vi "PB-01 Write.vi"(0 "Device Inputs":dbl[](array[numeric]), 12 "PB-01 in":T1={"FIFO Indexes"={"Write"={"Clear Faults"=0, "ESTTL Setup"=[], "UEGO Control"={"UEGO1Enable"=-1, "UEGO2Enable"=-1, "UEGO1Range"=-1, "UEGO2Range"=-1, "FilterCutoff (Hz)"=-1}}, "Read"={"UEGO Sensor Results"={"UEGO1Lambda"=-1, "UEGO1Phi"=-1, "UEGO1AFRatio"=-1, "UEGO1Ip (mA)"=-1, "UEGO2Lambda"=-1, "UEGO2Phi"=-1, "UEGO2AFRatio"=-1, "UEGO2Ip (mA)"=-1}, "UEGO Temperature (C)"={"UEGO1Temp (C)"=-1, "UEGO2Temp (C)"=-1, "UEGO1Hot"=-1, "UEGO2Hot"=-1}, "UEGO Diagnostics"={"UEGO1SensorFault"=-1, "UEGO2SensorFault"=-1, "UEGO1HeaterFault"=-1, "UEGO2HeaterFault"=-1, "UEGOFuseStatus"=-1, "Battery (V)"=-1, "LSUType"=-1}}}, "Settings"={"VR-Hall Mode Select"=[enum."VR Adaptive Arm", enum."VR Adaptive Arm", enum."VR Adaptive Arm", enum."VR Adaptive Arm", enum."VR Adaptive Arm"], "VR-Hall Arming Threshold [V]"=[0.0, 0.0, 0.0, 0.0, 0.0], "ESTTL Command Enabled"=FALSE}} {"FIFO Indexes"."Read"."UEGO Diagnostics"."LSUType" format="%02.0f"; "FIFO Indexes"."Read"."UEGO Diagnostics"."UEGOFuseStatus" format="%02.0f"}) -> (4 "VR-Hall Mode Select":T3[](array[typedef])=[enum."VR Adaptive Arm", enum."VR Adaptive Arm", enum."VR Adaptive Arm", enum."VR Adaptive Arm", enum."VR Adaptive Arm"], 6 "VR-Hall Arming/Threshold [V]":dbl[](array[numeric]), 8 "SensorControl":T7={"UEGO1Enable"=FALSE, "UEGO2Enable"=FALSE, "UEGO1Range"=FALSE, "UEGO2Range"=FALSE, "FilterCutoff (Hz)"=10.0}, 10 "Clear Faults":bool, 15 "ESTTL Setup":T4[](array[typedef])=[{"Mode"=enum."Off", "Polarity"=FALSE, "Frequency [Hz]"=0.0, "Duty Cycle [%]"=0.0, "TDC Offset [CAD]"=0.0, "Window Start [DBTDC]"=0.0, "Window End [DBTDC]"=0.0, "Angles"=[{"Enable"=FALSE, "Location [DBTDC]"=0.0, "Duration [s]"=0.0}, {"Enable"=FALSE, "Location [DBTDC]"=0.0, "Duration [s]"=0.0}, {"Enable"=FALSE, "Location [DBTDC]"=0.0, "Duration [s]"=0.0}, {"Enable"=FALSE, "Location [DBTDC]"=0.0, "Duration [s]"=0.0}], "Skip Fire"=FALSE, "Skip Fire Index"=0}, {"Mode"=enum."Off", "Polarity"=FALSE, "Frequency [Hz]"=0.0, "Duty Cycle [%]"=0.0, "TDC Offset [CAD]"=0.0, "Window Start [DBTDC]"=0.0, "Window End [DBTDC]"=0.0, "Angles"=[{"Enable"=FALSE, "Location [DBTDC]"=0.0, "Duration [s]"=0.0}, {"Enable"=FALSE, "Location [DBTDC]"=0.0, "Duration [s]"=0.0}, {"Enable"=FALSE, "Location [DBTDC]"=0.0, "Duration [s]"=0.0}, {"Enable"=FALSE, "Location [DBTDC]"=0.0, "Duration [s]"=0.0}], "Skip Fire"=FALSE, "Skip Fire Index"=0}, {"Mode"=enum."Off", "Polarity"=FALSE, "Frequency [Hz]"=0.0, "Duty Cycle [%]"=0.0, "TDC Offset [CAD]"=0.0, "Window Start [DBTDC]"=0.0, "Window End [DBTDC]"=0.0, "Angles"=[{"Enable"=FALSE, "Location [DBTDC]"=0.0, "Duration [s]"=0.0}, {"Enable"=FALSE, "Location [DBTDC]"=0.0, "Duration [s]"=0.0}, {"Enable"=FALSE, "Location [DBTDC]"=0.0, "Duration [s]"=0.0}, {"Enable"=FALSE, "Location [DBTDC]"=0.0, "Duration [s]"=0.0}], "Skip Fire"=FALSE, "Skip Fire Index"=0}, {"Mode"=enum."Off", "Polarity"=FALSE, "Frequency [Hz]"=0.0, "Duty Cycle [%]"=0.0, "TDC Offset [CAD]"=0.0, "Window Start [DBTDC]"=0.0, "Window End [DBTDC]"=0.0, "Angles"=[{"Enable"=FALSE, "Location [DBTDC]"=0.0, "Duration [s]"=0.0}, {"Enable"=FALSE, "Location [DBTDC]"=0.0, "Duration [s]"=0.0}, {"Enable"=FALSE, "Location [DBTDC]"=0.0, "Duration [s]"=0.0}, {"Enable"=FALSE, "Location [DBTDC]"=0.0, "Duration [s]"=0.0}], "Skip Fire"=FALSE, "Skip Fire Index"=0}, {"Mode"=enum."Off", "Polarity"=FALSE, "Frequency [Hz]"=0.0, "Duty Cycle [%]"=0.0, "TDC Offset [CAD]"=0.0, "Window Start [DBTDC]"=0.0, "Window End [DBTDC]"=0.0, "Angles"=[{"Enable"=FALSE, "Location [DBTDC]"=0.0, "Duration [s]"=0.0}, {"Enable"=FALSE, "Location [DBTDC]"=0.0, "Duration [s]"=0.0}, {"Enable"=FALSE, "Location [DBTDC]"=0.0, "Duration [s]"=0.0}, {"Enable"=FALSE, "Location [DBTDC]"=0.0, "Duration [s]"=0.0}], "Skip Fire"=FALSE, "Skip Fire Index"=0}, {"Mode"=enum."Off", "Polarity"=FALSE, "Frequency [Hz]"=0.0, "Duty Cycle [%]"=0.0, "TDC Offset [CAD]"=0.0, "Window Start [DBTDC]"=0.0, "Window End [DBTDC]"=0.0, "Angles"=[{"Enable"=FALSE, "Location [DBTDC]"=0.0, "Duration [s]"=0.0}, {"Enable"=FALSE, "Location [DBTDC]"=0.0, "Duration [s]"=0.0}, {"Enable"=FALSE, "Location [DBTDC]"=0.0, "Duration [s]"=0.0}, {"Enable"=FALSE, "Location [DBTDC]"=0.0, "Duration [s]"=0.0}], "Skip Fire"=FALSE, "Skip Fire Index"=0}, {"Mode"=enum."Off", "Polarity"=FALSE, "Frequency [Hz]"=0.0, "Duty Cycle [%]"=0.0, "TDC Offset [CAD]"=0.0, "Window Start [DBTDC]"=0.0, "Window End [DBTDC]"=0.0, "Angles"=[{"Enable"=FALSE, "Location [DBTDC]"=0.0, "Duration [s]"=0.0}, {"Enable"=FALSE, "Location [DBTDC]"=0.0, "Duration [s]"=0.0}, {"Enable"=FALSE, "Location [DBTDC]"=0.0, "Duration [s]"=0.0}, {"Enable"=FALSE, "Location [DBTDC]"=0.0, "Duration [s]"=0.0}], "Skip Fire"=FALSE, "Skip Fire Index"=0}, {"Mode"=enum."Off", "Polarity"=FALSE, "Frequency [Hz]"=0.0, "Duty Cycle [%]"=0.0, "TDC Offset [CAD]"=0.0, "Window Start [DBTDC]"=0.0, "Window End [DBTDC]"=0.0, "Angles"=[{"Enable"=FALSE, "Location [DBTDC]"=0.0, "Duration [s]"=0.0}, {"Enable"=FALSE, "Location [DBTDC]"=0.0, "Duration [s]"=0.0}, {"Enable"=FALSE, "Location [DBTDC]"=0.0, "Duration [s]"=0.0}, {"Enable"=FALSE, "Location [DBTDC]"=0.0, "Duration [s]"=0.0}], "Skip Fire"=FALSE, "Skip Fire Index"=0}, {"Mode"=enum."Off", "Polarity"=FALSE, "Frequency [Hz]"=0.0, "Duty Cycle [%]"=0.0, "TDC Offset [CAD]"=0.0, "Window Start [DBTDC]"=0.0, "Window End [DBTDC]"=0.0, "Angles"=[{"Enable"=FALSE, "Location [DBTDC]"=0.0, "Duration [s]"=0.0}, {"Enable"=FALSE, "Location [DBTDC]"=0.0, "Duration [s]"=0.0}, {"Enable"=FALSE, "Location [DBTDC]"=0.0, "Duration [s]"=0.0}, {"Enable"=FALSE, "Location [DBTDC]"=0.0, "Duration [s]"=0.0}], "Skip Fire"=FALSE, "Skip Fire Index"=0}, {"Mode"=enum."Off", "Polarity"=FALSE, "Frequency [Hz]"=0.0, "Duty Cycle [%]"=0.0, "TDC Offset [CAD]"=0.0, "Window Start [DBTDC]"=0.0, "Window End [DBTDC]"=0.0, "Angles"=[{"Enable"=FALSE, "Location [DBTDC]"=0.0, "Duration [s]"=0.0}, {"Enable"=FALSE, "Location [DBTDC]"=0.0, "Duration [s]"=0.0}, {"Enable"=FALSE, "Location [DBTDC]"=0.0, "Duration [s]"=0.0}, {"Enable"=FALSE, "Location [DBTDC]"=0.0, "Duration [s]"=0.0}], "Skip Fire"=FALSE, "Skip Fire Index"=0}, {"Mode"=enum."Off", "Polarity"=FALSE, "Frequency [Hz]"=0.0, "Duty Cycle [%]"=0.0, "TDC Offset [CAD]"=0.0, "Window Start [DBTDC]"=0.0, "Window End [DBTDC]"=0.0, "Angles"=[{"Enable"=FALSE, "Location [DBTDC]"=0.0, "Duration [s]"=0.0}, {"Enable"=FALSE, "Location [DBTDC]"=0.0, "Duration [s]"=0.0}, {"Enable"=FALSE, "Location [DBTDC]"=0.0, "Duration [s]"=0.0}, {"Enable"=FALSE, "Location [DBTDC]"=0.0, "Duration [s]"=0.0}], "Skip Fire"=FALSE, "Skip Fire Index"=0}, {"Mode"=enum."Off", "Polarity"=FALSE, "Frequency [Hz]"=0.0, "Duty Cycle [%]"=0.0, "TDC Offset [CAD]"=0.0, "Window Start [DBTDC]"=0.0, "Window End [DBTDC]"=0.0, "Angles"=[{"Enable"=FALSE, "Location [DBTDC]"=0.0, "Duration [s]"=0.0}, {"Enable"=FALSE, "Location [DBTDC]"=0.0, "Duration [s]"=0.0}, {"Enable"=FALSE, "Location [DBTDC]"=0.0, "Duration [s]"=0.0}, {"Enable"=FALSE, "Location [DBTDC]"=0.0, "Duration [s]"=0.0}], "Skip Fire"=FALSE, "Skip Fire Index"=0}, {"Mode"=enum."Off", "Polarity"=FALSE, "Frequency [Hz]"=0.0, "Duty Cycle [%]"=0.0, "TDC Offset [CAD]"=0.0, "Window Start [DBTDC]"=0.0, "Window End [DBTDC]"=0.0, "Angles"=[{"Enable"=FALSE, "Location [DBTDC]"=0.0, "Duration [s]"=0.0}, {"Enable"=FALSE, "Location [DBTDC]"=0.0, "Duration [s]"=0.0}, {"Enable"=FALSE, "Location [DBTDC]"=0.0, "Duration [s]"=0.0}, {"Enable"=FALSE, "Location [DBTDC]"=0.0, "Duration [s]"=0.0}], "Skip Fire"=FALSE, "Skip Fire Index"=0}, {"Mode"=enum."Off", "Polarity"=FALSE, "Frequency [Hz]"=0.0, "Duty Cycle [%]"=0.0, "TDC Offset [CAD]"=0.0, "Window Start [DBTDC]"=0.0, "Window End [DBTDC]"=0.0, "Angles"=[{"Enable"=FALSE, "Location [DBTDC]"=0.0, "Duration [s]"=0.0}, {"Enable"=FALSE, "Location [DBTDC]"=0.0, "Duration [s]"=0.0}, {"Enable"=FALSE, "Location [DBTDC]"=0.0, "Duration [s]"=0.0}, {"Enable"=FALSE, "Location [DBTDC]"=0.0, "Duration [s]"=0.0}], "Skip Fire"=FALSE, "Skip Fire Index"=0}, {"Mode"=enum."Off", "Polarity"=FALSE, "Frequency [Hz]"=0.0, "Duty Cycle [%]"=0.0, "TDC Offset [CAD]"=0.0, "Window Start [DBTDC]"=0.0, "Window End [DBTDC]"=0.0, "Angles"=[{"Enable"=FALSE, "Location [DBTDC]"=0.0, "Duration [s]"=0.0}, {"Enable"=FALSE, "Location [DBTDC]"=0.0, "Duration [s]"=0.0}, {"Enable"=FALSE, "Location [DBTDC]"=0.0, "Duration [s]"=0.0}, {"Enable"=FALSE, "Location [DBTDC]"=0.0, "Duration [s]"=0.0}], "Skip Fire"=FALSE, "Skip Fire Index"=0}, {"Mode"=enum."Off", "Polarity"=FALSE, "Frequency [Hz]"=0.0, "Duty Cycle [%]"=0.0, "TDC Offset [CAD]"=0.0, "Window Start [DBTDC]"=0.0, "Window End [DBTDC]"=0.0, "Angles"=[{"Enable"=FALSE, "Location [DBTDC]"=0.0, "Duration [s]"=0.0}, {"Enable"=FALSE, "Location [DBTDC]"=0.0, "Duration [s]"=0.0}, {"Enable"=FALSE, "Location [DBTDC]"=0.0, "Duration [s]"=0.0}, {"Enable"=FALSE, "Location [DBTDC]"=0.0, "Duration [s]"=0.0}], "Skip Fire"=FALSE, "Skip Fire Index"=0}] {"Skip Fire Index" max=7; "Angles"."Duration [s]" format="%#_3p"; "Frequency [Hz]" format="%#_3p"})   [LabVIEW 2015]
uses:
  <vilib>/Powertrain Controls/Device Drivers/VR-Hall/RevC/Real-Time/Support/Vr_Hall_mode_control_revc.ctl
  <vilib>/Powertrain Controls/Device Drivers/DCM/ESTTL/RT/Setup.ctl
  <vilib>/Powertrain Controls/Device Drivers/DCM/ESTTL/FPGA/Mode.ctl
  <vilib>/Powertrain Controls/Device Drivers/DCM/ESTTL/RT/Angle Control.ctl
  DCM-NIVS-RT/PB-01.ctl
  DCM-NIVS-RT/ESTTL Setup Indexes.ctl
  <vilib>/Powertrain Controls/Device Drivers/DCM/ESTTL/RT/DCM - RT - ESTTL.lvlib
  <vilib>/Powertrain Controls/Device Drivers/DCM/ESTTL/FPGA/DCM - FPGA - ESTTL.lvlib
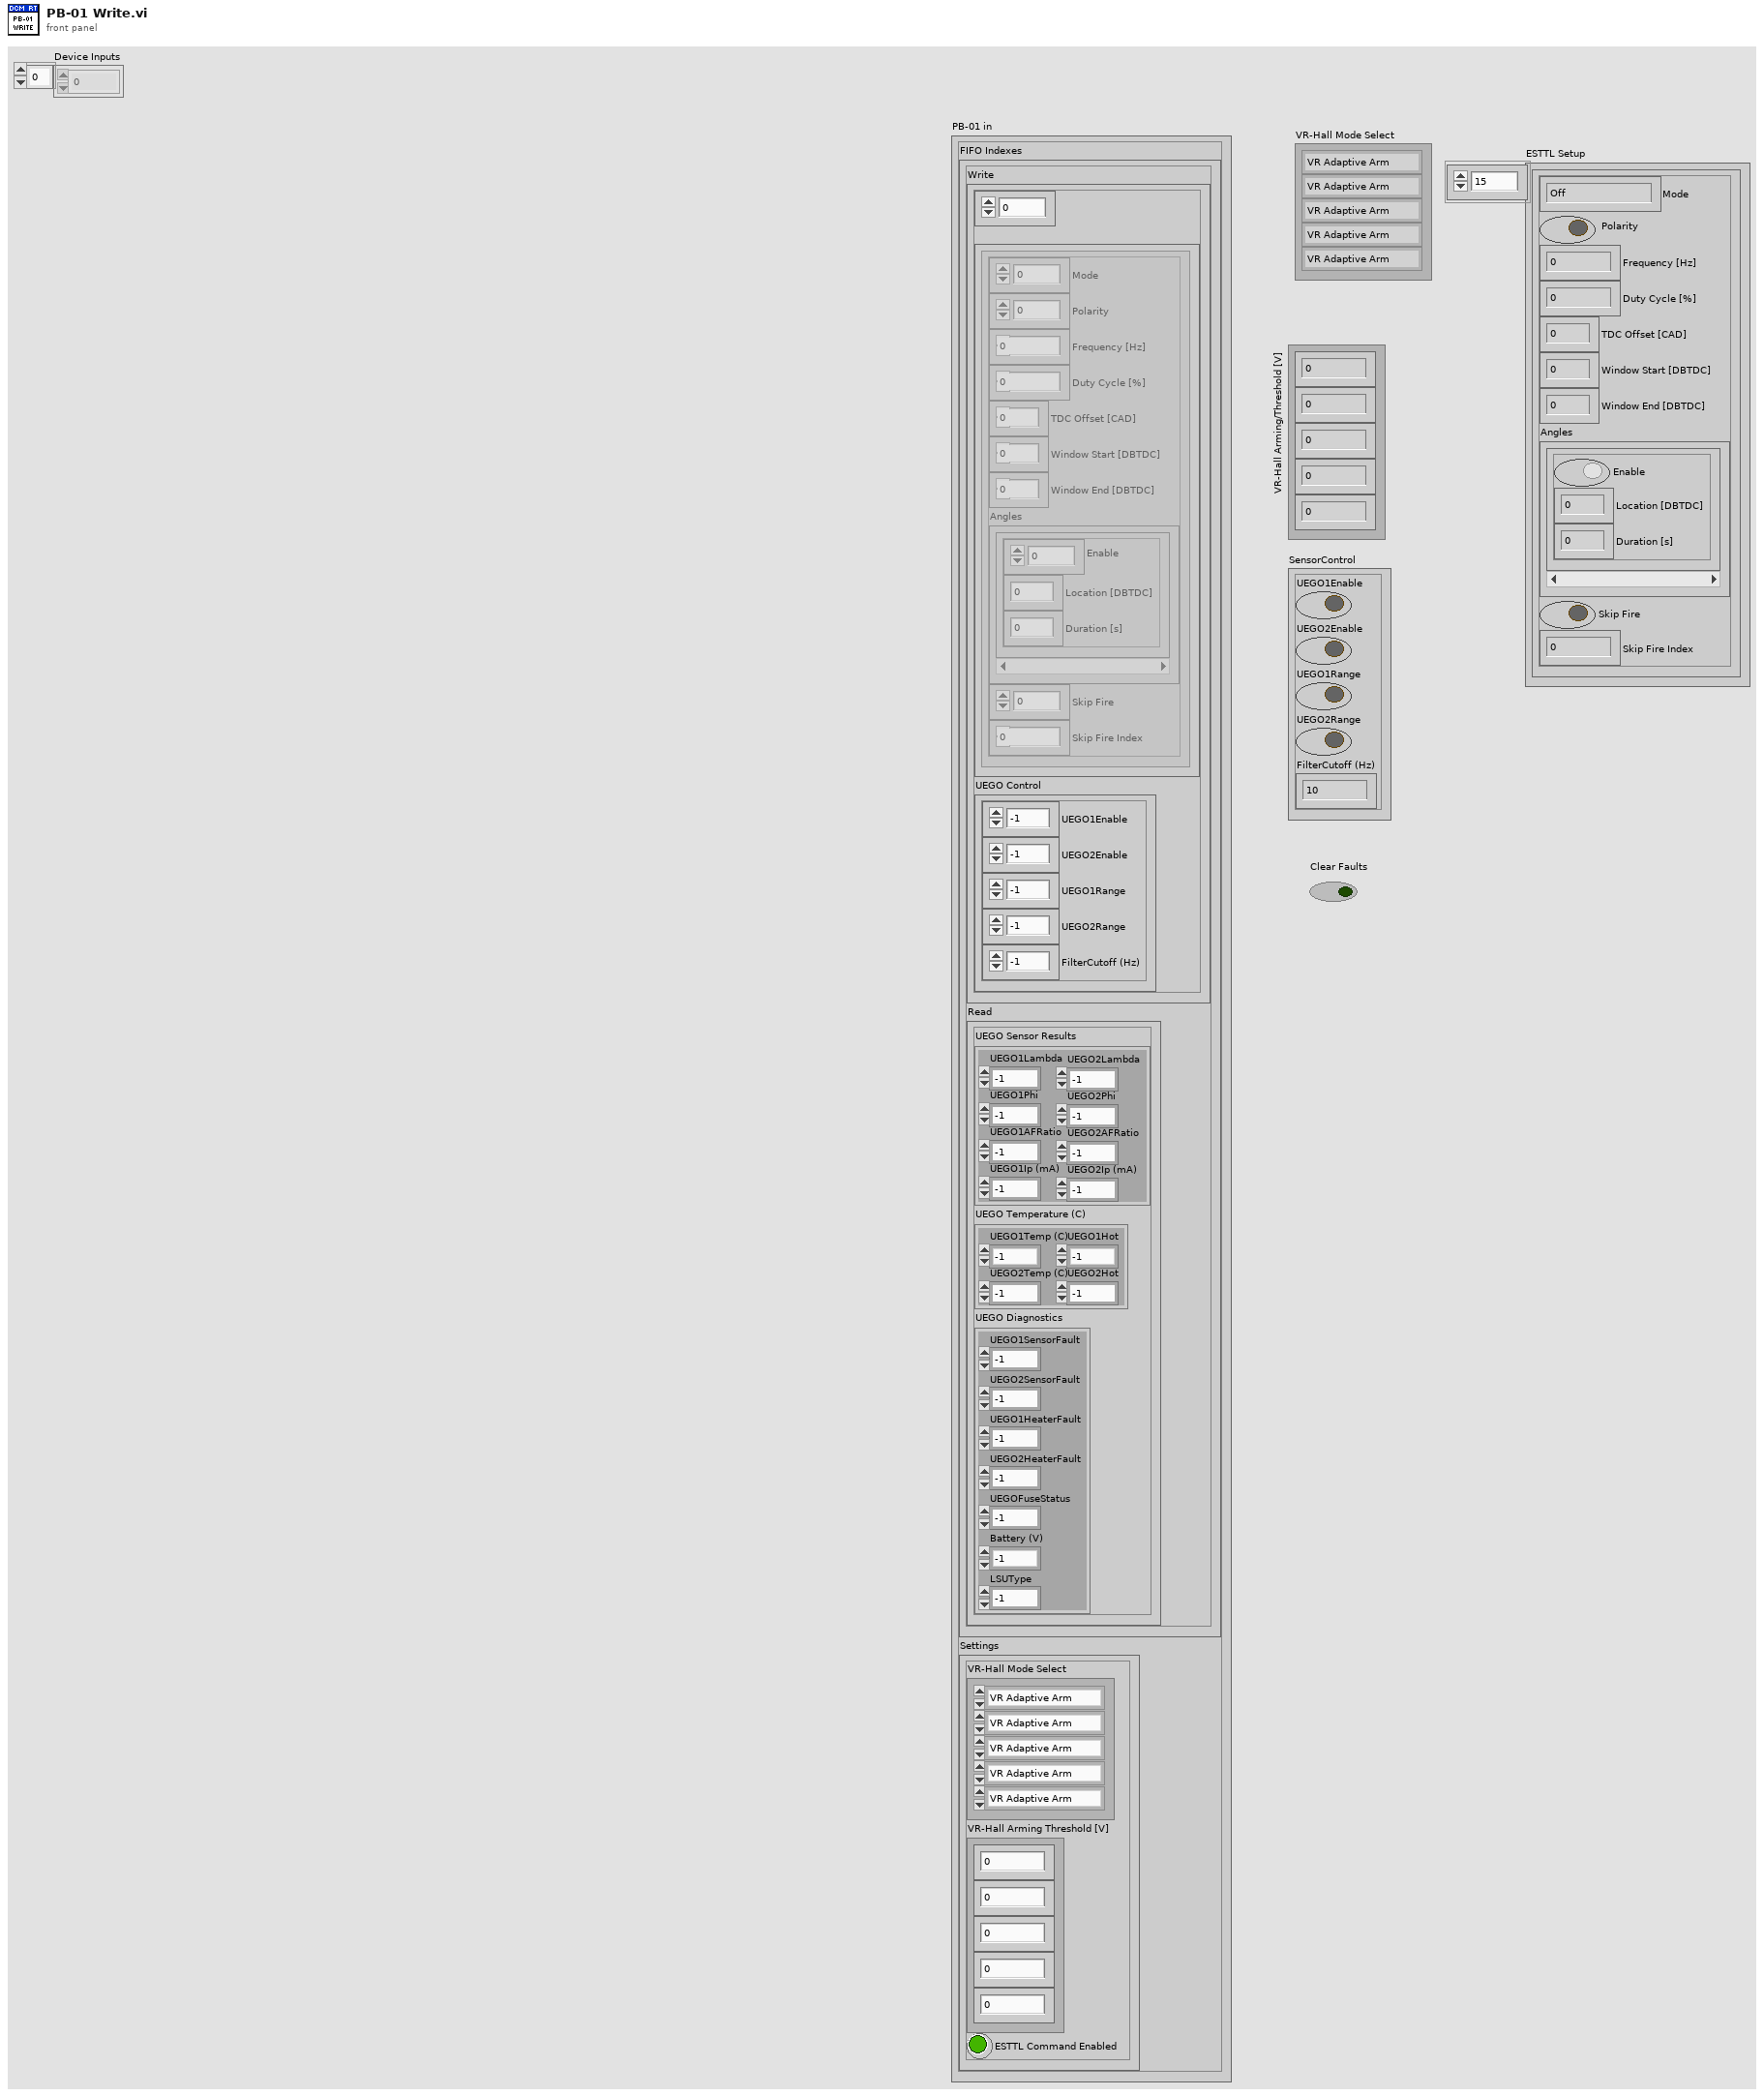
[diagram p1: front panel]
types:
  T1 = typedef "PB-01.ctl" = cluster{"FIFO Indexes":cluster{"Write":cluster{"Clear Faults":i32, "ESTTL Setup":T2[], "UEGO Control":cluster{"UEGO1Enable":i32, "UEGO2Enable":i32, "UEGO1Range":i32, "UEGO2Range":i32, "FilterCutoff (Hz)":i32}}, "Read":cluster{"UEGO Sensor Results":cluster{"UEGO1Lambda":i32, "UEGO1Phi":i32, "UEGO1AFRatio":i32, "UEGO1Ip (mA)":i32, "UEGO2Lambda":i32, "UEGO2Phi":i32, "UEGO2AFRatio":i32, "UEGO2Ip (mA)":i32}, "UEGO Temperature (C)":cluster{"UEGO1Temp (C)":i32, "UEGO2Temp (C)":i32, "UEGO1Hot":i32, "UEGO2Hot":i32}, "UEGO Diagnostics":cluster{"UEGO1SensorFault":i32, "UEGO2SensorFault":i32, "UEGO1HeaterFault":i32, "UEGO2HeaterFault":i32, "UEGOFuseStatus":i32, "Battery (V)":i32, "LSUType":i32}}}, "Settings":cluster{"VR-Hall Mode Select":T3[], "VR-Hall Arming Threshold [V]":dbl[], "ESTTL Command Enabled":bool}}
  T2 = typedef "ESTTL Setup Indexes.ctl" = cluster{"Mode":i32, "Polarity":i32, "Frequency [Hz]":i32, "Duty Cycle [%]":i32, "TDC Offset [CAD]":i32, "Window Start [DBTDC]":i32, "Window End [DBTDC]":i32, "Angles":cluster{"Enable":i32, "Location [DBTDC]":i32, "Duration [s]":i32}[], "Skip Fire":i32, "Skip Fire Index":i32}
  T3 = typedef "Vr_Hall_mode_control_revc.ctl" = enum32{"VR Adaptive Arm", "VR Manual Arm", "Hall", "Hall w/ Pull-up"}
  T4 = typedef "DCM - RT - ESTTL.lvlib/Setup.ctl" = cluster{"Mode":T5, "Polarity":bool, "Frequency [Hz]":sgl, "Duty Cycle [%]":sgl, "TDC Offset [CAD]":sgl, "Window Start [DBTDC]":sgl, "Window End [DBTDC]":sgl, "Angles":T6[], "Skip Fire":bool, "Skip Fire Index":u8}
  T5 = typedef "DCM - FPGA - ESTTL.lvlib/Mode.ctl" = enum8{"Off", "Pulse Width Modulation", "Engine Position Tracking"}
  T6 = typedef "DCM - RT - ESTTL.lvlib/Angle Control.ctl" = cluster{"Enable":bool, "Location [DBTDC]":sgl, "Duration [s]":sgl}
  T7 = cluster{"UEGO1Enable":bool, "UEGO2Enable":bool, "UEGO1Range":bool, "UEGO2Range":bool, "FilterCutoff (Hz)":dbl}
  T8 = cluster{"UEGO1Enable":i32, "UEGO2Enable":i32, "UEGO1Range":i32, "UEGO2Range":i32, "FilterCutoff (Hz)":i32}
  T9 = cluster{"Enable":i32, "Location [DBTDC]":i32, "Duration [s]":i32}[]
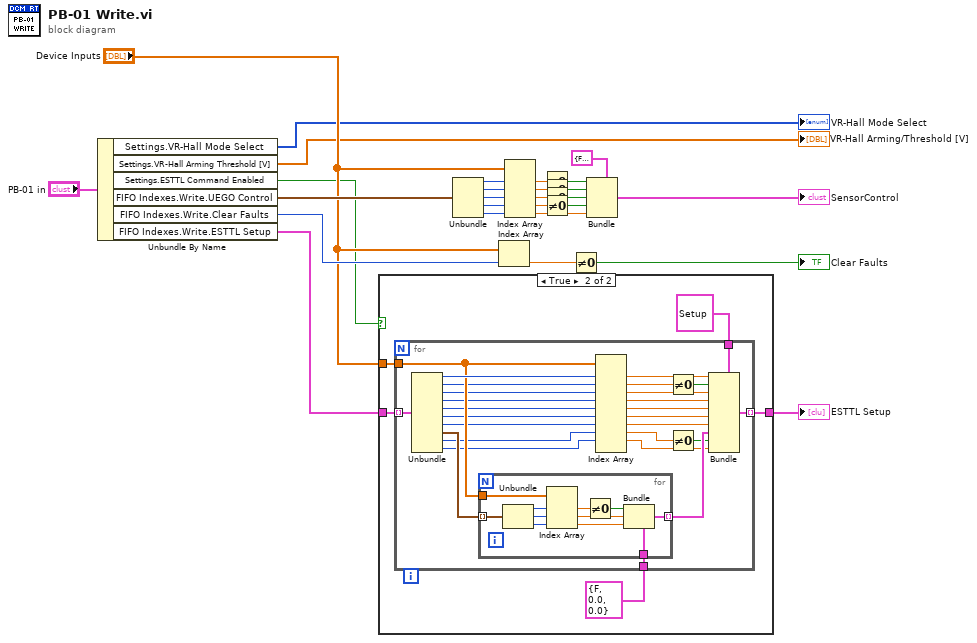
[diagram p0: block diagram]
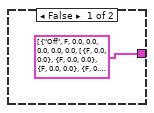
[diagram p2: hidden frame]
diagram:
  n1 = Unbundle By Name("PB-01 in") -> ("Settings.VR-Hall Mode Select"=→"VR-Hall Mode Select":T3[], "Settings.VR-Hall Arming Threshold [V]"=→"VR-Hall Arming/Threshold [V]":dbl[], "Settings.ESTTL Command Enabled"=w1:bool, "FIFO Indexes.Write.UEGO Control"=w23:T8, "FIFO Indexes.Write.Clear Faults"=w26:i32, "FIFO Indexes.Write.ESTTL Setup"=w27:T2[])
  n2 = case shown="True" w1 {
    tunnel: w27 -> [_ w33]
    tunnel: [T4[] [{"Mode"=enum."Off", "Polarity"=FALSE, "Frequency [Hz]"=0.0, "Duty Cycle [%]"=0.0, "TDC Offset [CAD]"=0.0, "Window Start [DBTDC]"=0.0, "Window End [DBTDC]"=0.0, "Angles"=[{"Enable"=FALSE, "Location [DBTDC]"=0.0, "Duration [s]"=0.0}, {"Enable"=FALSE, "Location [DBTDC]"=0.0, "Duration [s]"=0.0}, {"Enable"=FALSE, "Location [DBTDC]"=0.0, "Duration [s]"=0.0}, {"Enable"=FALSE, "Location [DBTDC]"=0.0, "Duration [s]"=0.0}], "Skip Fire"=FALSE, "Skip Fire Index"=0}, {"Mode"=enum."Off", "Polarity"=FALSE, "Frequency [Hz]"=0.0, "Duty Cycle [%]"=0.0, "TDC Offset [CAD]"=0.0, "Window Start [DBTDC]"=0.0, "Window End [DBTDC]"=0.0, "Angles"=[{"Enable"=FALSE, "Location [DBTDC]"=0.0, "Duration [s]"=0.0}, {"Enable"=FALSE, "Location [DBTDC]"=0.0, "Duration [s]"=0.0}, {"Enable"=FALSE, "Location [DBTDC]"=0.0, "Duration [s]"=0.0}, {"Enable"=FALSE, "Location [DBTDC]"=0.0, "Duration [s]"=0.0}], "Skip Fire"=FALSE, "Skip Fire Index"=0}, {"Mode"=enum."Off", "Polarity"=FALSE, "Frequency [Hz]"=0.0, "Duty Cycle [%]"=0.0, "TDC Offset [CAD]"=0.0, "Window Start [DBTDC]"=0.0, "Window End [DBTDC]"=0.0, "Angles"=[{"Enable"=FALSE, "Location [DBTDC]"=0.0, "Duration [s]"=0.0}, {"Enable"=FALSE, "Location [DBTDC]"=0.0, "Duration [s]"=0.0}, {"Enable"=FALSE, "Location [DBTDC]"=0.0, "Duration [s]"=0.0}, {"Enable"=FALSE, "Location [DBTDC]"=0.0, "Duration [s]"=0.0}], "Skip Fire"=FALSE, "Skip Fire Index"=0}, {"Mode"=enum."Off", "Polarity"=FALSE, "Frequency [Hz]"=0.0, "Duty Cycle [%]"=0.0, "TDC Offset [CAD]"=0.0, "Window Start [DBTDC]"=0.0, "Window End [DBTDC]"=0.0, "Angles"=[{"Enable"=FALSE, "Location [DBTDC]"=0.0, "Duration [s]"=0.0}, {"Enable"=FALSE, "Location [DBTDC]"=0.0, "Duration [s]"=0.0}, {"Enable"=FALSE, "Location [DBTDC]"=0.0, "Duration [s]"=0.0}, {"Enable"=FALSE, "Location [DBTDC]"=0.0, "Duration [s]"=0.0}], "Skip Fire"=FALSE, "Skip Fire Index"=0}, {"Mode"=enum."Off", "Polarity"=FALSE, "Frequency [Hz]"=0.0, "Duty Cycle [%]"=0.0, "TDC Offset [CAD]"=0.0, "Window Start [DBTDC]"=0.0, "Window End [DBTDC]"=0.0, "Angles"=[{"Enable"=FALSE, "Location [DBTDC]"=0.0, "Duration [s]"=0.0}, {"Enable"=FALSE, "Location [DBTDC]"=0.0, "Duration [s]"=0.0}, {"Enable"=FALSE, "Location [DBTDC]"=0.0, "Duration [s]"=0.0}, {"Enable"=FALSE, "Location [DBTDC]"=0.0, "Duration [s]"=0.0}], "Skip Fire"=FALSE, "Skip Fire Index"=0}, {"Mode"=enum."Off", "Polarity"=FALSE, "Frequency [Hz]"=0.0, "Duty Cycle [%]"=0.0, "TDC Offset [CAD]"=0.0, "Window Start [DBTDC]"=0.0, "Window End [DBTDC]"=0.0, "Angles"=[{"Enable"=FALSE, "Location [DBTDC]"=0.0, "Duration [s]"=0.0}, {"Enable"=FALSE, "Location [DBTDC]"=0.0, "Duration [s]"=0.0}, {"Enable"=FALSE, "Location [DBTDC]"=0.0, "Duration [s]"=0.0}, {"Enable"=FALSE, "Location [DBTDC]"=0.0, "Duration [s]"=0.0}], "Skip Fire"=FALSE, "Skip Fire Index"=0}, {"Mode"=enum."Off", "Polarity"=FALSE, "Frequency [Hz]"=0.0, "Duty Cycle [%]"=0.0, "TDC Offset [CAD]"=0.0, "Window Start [DBTDC]"=0.0, "Window End [DBTDC]"=0.0, "Angles"=[{"Enable"=FALSE, "Location [DBTDC]"=0.0, "Duration [s]"=0.0}, {"Enable"=FALSE, "Location [DBTDC]"=0.0, "Duration [s]"=0.0}, {"Enable"=FALSE, "Location [DBTDC]"=0.0, "Duration [s]"=0.0}, {"Enable"=FALSE, "Location [DBTDC]"=0.0, "Duration [s]"=0.0}], "Skip Fire"=FALSE, "Skip Fire Index"=0}, {"Mode"=enum."Off", "Polarity"=FALSE, "Frequency [Hz]"=0.0, "Duty Cycle [%]"=0.0, "TDC Offset [CAD]"=0.0, "Window Start [DBTDC]"=0.0, "Window End [DBTDC]"=0.0, "Angles"=[{"Enable"=FALSE, "Location [DBTDC]"=0.0, "Duration [s]"=0.0}, {"Enable"=FALSE, "Location [DBTDC]"=0.0, "Duration [s]"=0.0}, {"Enable"=FALSE, "Location [DBTDC]"=0.0, "Duration [s]"=0.0}, {"Enable"=FALSE, "Location [DBTDC]"=0.0, "Duration [s]"=0.0}], "Skip Fire"=FALSE, "Skip Fire Index"=0}, {"Mode"=enum."Off", "Polarity"=FALSE, "Frequency [Hz]"=0.0, "Duty Cycle [%]"=0.0, "TDC Offset [CAD]"=0.0, "Window Start [DBTDC]"=0.0, "Window End [DBTDC]"=0.0, "Angles"=[{"Enable"=FALSE, "Location [DBTDC]"=0.0, "Duration [s]"=0.0}, {"Enable"=FALSE, "Location [DBTDC]"=0.0, "Duration [s]"=0.0}, {"Enable"=FALSE, "Location [DBTDC]"=0.0, "Duration [s]"=0.0}, {"Enable"=FALSE, "Location [DBTDC]"=0.0, "Duration [s]"=0.0}], "Skip Fire"=FALSE, "Skip Fire Index"=0}, {"Mode"=enum."Off", "Polarity"=FALSE, "Frequency [Hz]"=0.0, "Duty Cycle [%]"=0.0, "TDC Offset [CAD]"=0.0, "Window Start [DBTDC]"=0.0, "Window End [DBTDC]"=0.0, "Angles"=[{"Enable"=FALSE, "Location [DBTDC]"=0.0, "Duration [s]"=0.0}, {"Enable"=FALSE, "Location [DBTDC]"=0.0, "Duration [s]"=0.0}, {"Enable"=FALSE, "Location [DBTDC]"=0.0, "Duration [s]"=0.0}, {"Enable"=FALSE, "Location [DBTDC]"=0.0, "Duration [s]"=0.0}], "Skip Fire"=FALSE, "Skip Fire Index"=0}, {"Mode"=enum."Off", "Polarity"=FALSE, "Frequency [Hz]"=0.0, "Duty Cycle [%]"=0.0, "TDC Offset [CAD]"=0.0, "Window Start [DBTDC]"=0.0, "Window End [DBTDC]"=0.0, "Angles"=[{"Enable"=FALSE, "Location [DBTDC]"=0.0, "Duration [s]"=0.0}, {"Enable"=FALSE, "Location [DBTDC]"=0.0, "Duration [s]"=0.0}, {"Enable"=FALSE, "Location [DBTDC]"=0.0, "Duration [s]"=0.0}, {"Enable"=FALSE, "Location [DBTDC]"=0.0, "Duration [s]"=0.0}], "Skip Fire"=FALSE, "Skip Fire Index"=0}, {"Mode"=enum."Off", "Polarity"=FALSE, "Frequency [Hz]"=0.0, "Duty Cycle [%]"=0.0, "TDC Offset [CAD]"=0.0, "Window Start [DBTDC]"=0.0, "Window End [DBTDC]"=0.0, "Angles"=[{"Enable"=FALSE, "Location [DBTDC]"=0.0, "Duration [s]"=0.0}, {"Enable"=FALSE, "Location [DBTDC]"=0.0, "Duration [s]"=0.0}, {"Enable"=FALSE, "Location [DBTDC]"=0.0, "Duration [s]"=0.0}, {"Enable"=FALSE, "Location [DBTDC]"=0.0, "Duration [s]"=0.0}], "Skip Fire"=FALSE, "Skip Fire Index"=0}, {"Mode"=enum."Off", "Polarity"=FALSE, "Frequency [Hz]"=0.0, "Duty Cycle [%]"=0.0, "TDC Offset [CAD]"=0.0, "Window Start [DBTDC]"=0.0, "Window End [DBTDC]"=0.0, "Angles"=[{"Enable"=FALSE, "Location [DBTDC]"=0.0, "Duration [s]"=0.0}, {"Enable"=FALSE, "Location [DBTDC]"=0.0, "Duration [s]"=0.0}, {"Enable"=FALSE, "Location [DBTDC]"=0.0, "Duration [s]"=0.0}, {"Enable"=FALSE, "Location [DBTDC]"=0.0, "Duration [s]"=0.0}], "Skip Fire"=FALSE, "Skip Fire Index"=0}, {"Mode"=enum."Off", "Polarity"=FALSE, "Frequency [Hz]"=0.0, "Duty Cycle [%]"=0.0, "TDC Offset [CAD]"=0.0, "Window Start [DBTDC]"=0.0, "Window End [DBTDC]"=0.0, "Angles"=[{"Enable"=FALSE, "Location [DBTDC]"=0.0, "Duration [s]"=0.0}, {"Enable"=FALSE, "Location [DBTDC]"=0.0, "Duration [s]"=0.0}, {"Enable"=FALSE, "Location [DBTDC]"=0.0, "Duration [s]"=0.0}, {"Enable"=FALSE, "Location [DBTDC]"=0.0, "Duration [s]"=0.0}], "Skip Fire"=FALSE, "Skip Fire Index"=0}, {"Mode"=enum."Off", "Polarity"=FALSE, "Frequency [Hz]"=0.0, "Duty Cycle [%]"=0.0, "TDC Offset [CAD]"=0.0, "Window Start [DBTDC]"=0.0, "Window End [DBTDC]"=0.0, "Angles"=[{"Enable"=FALSE, "Location [DBTDC]"=0.0, "Duration [s]"=0.0}, {"Enable"=FALSE, "Location [DBTDC]"=0.0, "Duration [s]"=0.0}, {"Enable"=FALSE, "Location [DBTDC]"=0.0, "Duration [s]"=0.0}, {"Enable"=FALSE, "Location [DBTDC]"=0.0, "Duration [s]"=0.0}], "Skip Fire"=FALSE, "Skip Fire Index"=0}, {"Mode"=enum."Off", "Polarity"=FALSE, "Frequency [Hz]"=0.0, "Duty Cycle [%]"=0.0, "TDC Offset [CAD]"=0.0, "Window Start [DBTDC]"=0.0, "Window End [DBTDC]"=0.0, "Angles"=[{"Enable"=FALSE, "Location [DBTDC]"=0.0, "Duration [s]"=0.0}, {"Enable"=FALSE, "Location [DBTDC]"=0.0, "Duration [s]"=0.0}, {"Enable"=FALSE, "Location [DBTDC]"=0.0, "Duration [s]"=0.0}, {"Enable"=FALSE, "Location [DBTDC]"=0.0, "Duration [s]"=0.0}], "Skip Fire"=FALSE, "Skip Fire Index"=0}] ("ESTTL Setup") w30] -> w5
    tunnel: "Device Inputs" -> [_ w29]
    frame False {
    }
    frame True {
      n3 = for {
        tunnel: w33 -> [w60] mode=indexing
        tunnel: w29 -> [w57]
        tunnel: T6 {"Enable"=FALSE, "Location [DBTDC]"=0.0, "Duration [s]"=0.0} ("Injection Control") -> [w48]
        tunnel: T4 {"Mode"=enum."Off", "Polarity"=FALSE, "Frequency [Hz]"=0.0, "Duty Cycle [%]"=0.0, "TDC Offset [CAD]"=0.0, "Window Start [DBTDC]"=0.0, "Window End [DBTDC]"=0.0, "Angles"=[{"Enable"=FALSE, "Location [DBTDC]"=0.0, "Duration [s]"=0.0}, {"Enable"=FALSE, "Location [DBTDC]"=0.0, "Duration [s]"=0.0}, {"Enable"=FALSE, "Location [DBTDC]"=0.0, "Duration [s]"=0.0}, {"Enable"=FALSE, "Location [DBTDC]"=0.0, "Duration [s]"=0.0}], "Skip Fire"=FALSE, "Skip Fire Index"=0} ("DCM - RevB - RT - ESTTL.lvlib:Setup") -> [w35]
        tunnel: [w34] -> w30 mode=indexing
        n4 = Unbundle(w60) -> ("Mode"=w58:i32, "Polarity"=w56:i32, "Frequency [Hz]"=w55:i32, "Duty Cycle [%]"=w54:i32, "TDC Offset [CAD]"=w53:i32, "Window Start [DBTDC]"=w52:i32, "Window End [DBTDC]"=w51:i32, "Angles"=w59:T9, "Skip Fire"=w50:i32, "Skip Fire Index"=w49:i32)
        n5 = for {
          tunnel: w59 -> [w71] mode=indexing
          tunnel: w57 -> [w69]
          tunnel: w48 -> [w65]
          tunnel: [w61] -> w40 mode=indexing
          n6 = Unbundle(w71) -> ("Enable"=w70:i32, "Location [DBTDC]"=w68:i32, "Duration [s]"=w67:i32)
          n7 = Index Array(array=w69, index #1=w70, index #2=w68, index #3=w67) -> (element #1=w66:dbl, element #2=w64:dbl, element #3=w63:dbl)
          n8 = Not Equal To 0?(x=w66) -> (x != 0?=w62:bool)
          n9 = Bundle(cluster=w65, "Enable"=w62, "Location [DBTDC]"=w64, "Duration [s]"=w63) -> (w61:T6)
        }
        n10 = Index Array(array=w57, index #1=w58, index #2=w56, index #3=w55, index #4=w54, index #5=w53, index #6=w52, index #7=w51, index #8=w50, index #9=w49) -> (element #1=w47:dbl, element #2=w46:dbl, element #3=w45:dbl, element #4=w44:dbl, element #5=w43:dbl, element #6=w42:dbl, element #7=w41:dbl, element #8=w39:dbl, element #9=w38:dbl)  [unwired: 1 in, 1 out]
        n11 = Not Equal To 0?(x=w46) -> (x != 0?=w37:bool)
        n12 = Not Equal To 0?(x=w39) -> (x != 0?=w36:bool)
        n13 = Bundle(cluster=w35, "Mode"=w47, "Polarity"=w37, "Frequency [Hz]"=w45, "Duty Cycle [%]"=w44, "TDC Offset [CAD]"=w43, "Window Start [DBTDC]"=w42, "Window End [DBTDC]"=w41, "Angles"=w40, "Skip Fire"=w36, "Skip Fire Index"=w38) -> (w34:T4)
      }
    }
  }
  "ESTTL Setup" <- w5
  n14 = Unbundle(w23) -> ("UEGO1Enable"=w22:i32, "UEGO2Enable"=w21:i32, "UEGO1Range"=w20:i32, "UEGO2Range"=w19:i32, "FilterCutoff (Hz)"=w18:i32)
  n15 = Index Array(array="Device Inputs", index=w26) -> (element=w25:dbl)
  n16 = Index Array(array="Device Inputs", index #1=w22, index #2=w21, index #3=w20, index #4=w19, index #5=w18) -> (element #1=w17:dbl, element #2=w15:dbl, element #3=w16:dbl, element #4=w14:dbl, element #5=w8:dbl)
  n17 = Not Equal To 0?(x=w17) -> (x != 0?=w12:bool)
  n18 = Not Equal To 0?(x=w15) -> (x != 0?=w11:bool)
  n19 = Not Equal To 0?(x=w16) -> (x != 0?=w10:bool)
  n20 = Not Equal To 0?(x=w14) -> (x != 0?=w9:bool)
  n21 = Not Equal To 0?(x=w25) -> (x != 0?=→"Clear Faults":bool)
  n22 = Bundle(cluster=T7 {"UEGO1Enable"=FALSE, "UEGO2Enable"=FALSE, "UEGO1Range"=FALSE, "UEGO2Range"=FALSE, "FilterCutoff (Hz)"=10.0} ("SensorControl"), "UEGO1Enable"=w12, "UEGO2Enable"=w11, "UEGO1Range"=w10, "UEGO2Range"=w9, "FilterCutoff (Hz)"=w8) -> (→"SensorControl":T7)
